vi "RT Loop - RSI Low Speed.vi"(11 "Message Queue":refnum<queue>) -> ()   [LabVIEW 2018]
doc: "This RSI Low Speed Loop VI acquires temperature data and digital inputs, and updates digital outputs."
uses:
  support/Message Queue/Message Cluster.ctl
  <vilib>/Platform/TimedLoop/XDataNode/timing_clust.ctl
  <vilib>/Platform/TimedLoop/XDataNode/nitl_modes.ctl
  <vilib>/Platform/TimedLoop/XDataNode/wakeup.ctl
  controls/Control State.ctl
  <vilib>/Platform/TimedLoop/XDataNode/loadnilvce.vi
  <vilib>/Platform/TimedLoop/XDataNode/XDataNode.xnode
  <vilib>/Platform/TimedLoop/XDataNode/XDNodeRunTimeDep.lvlib
  support/Message Queue/Message Queue.lvlib
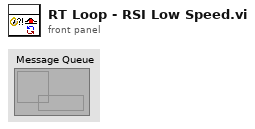
[diagram p1: front panel]
types:
  T1 = typedef "XDNodeRunTimeDep.lvlib/timing_clust.ctl" = cluster{"Expected End [f-1]":u64, "Actual End [f-1]":u64, "Finished Late? [f-1]":bool, "Expected End [i-1]":u64, "Actual End [i-1]":u64, "Finished Late? [i-1]":bool, "Expected Start [i]":u64, "Actual Start [i]":u64, "Expected Start [f]":u64, "Actual Start [f]":u64, "Source Name":string, "Structure Name":string, "Period":i64, "Deadline":i64, "Offset":i64, "Start":i64, "Priority":i32, "Timeout":i32, "Mode":T2, "Wakeup Reason":T3, "Error":errorcluster, "Source Type":string, "Secondary Source Type":string, "Global End Time":u64, "Global Start Time":u64, "Frame Duration":u64, "Iteration Duration":u64, "Assigned CPU":i32, "I/O Scan Engine Mode":u32}
  T2 = typedef "XDNodeRunTimeDep.lvlib/nitl_modes.ctl" = enum32{"No Change", "Process missed periods, maintain original phase", "Discard missed periods, maintain original phase", "Process missed periods, ignore original phase", "Discard missed periods, ignore original phase"}
  T3 = typedef "XDNodeRunTimeDep.lvlib/wakeup.ctl" = enum32{"Normal", "Aborted", "Asynchronous wakeup", "Timing source error", "Timed loop error", "Timeout"}
  T4 = typedef "Control State.ctl" = enum16{"Safe State", "Control (PID)"}
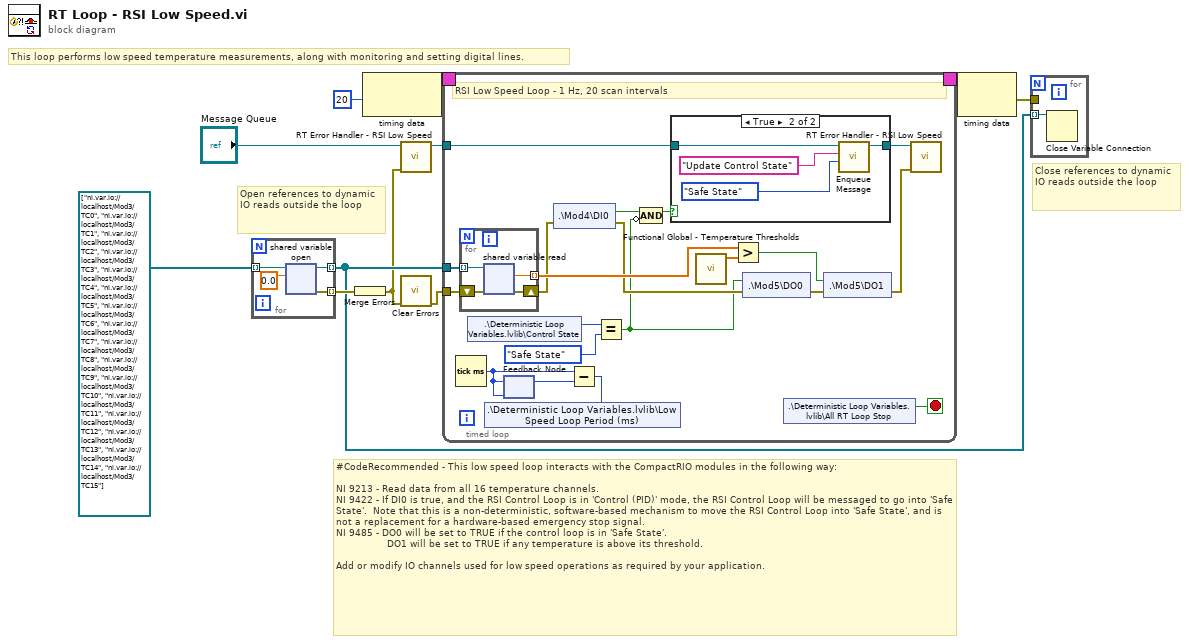
[diagram p0: block diagram]
diagram:
  # "Close references to dynamic IO reads outside the loop"
  # "Open references to dynamic IO reads outside the loop"
  # "#CodeRecommended - This low speed loop interacts with the CompactRIO modules in the following way:\n\nNI 9213 - Read data from all 16 temperature channels.\nNI 9422 - If DI0 is true, and the RSI Control Loop is in 'Control (PID)' mode, the RSI Control Loop will be messaged to go into 'Safe State'.  Note that this is a non-deterministic, software-based mechanism to move the RSI Control Loop into 'Safe State', and is not a replacement for a hardware-based emergency stop signal.\nNI 9485 - DO0 will be set to TRUE if the control loop is in 'Safe State'.\n                 DO1 will be set to TRUE if any temperature is above its threshold.\n\nAdd or modify IO channels used for low speed operations as required by your application."
  # "This loop performs low speed temperature measurements, along with monitoring and setting digital lines."
  n1 = for {
    tunnel: refnum<k21>[] ["ni.var.io://localhost/Mod3/TC0", "ni.var.io://localhost/Mod3/TC1", "ni.var.io://localhost/Mod3/TC2", "ni.var.io://localhost/Mod3/TC3", "ni.var.io://localhost/Mod3/TC4", "ni.var.io://localhost/Mod3/TC5", "ni.var.io://localhost/Mod3/TC6", "ni.var.io://localhost/Mod3/TC7", "ni.var.io://localhost/Mod3/TC8", "ni.var.io://localhost/Mod3/TC9", "ni.var.io://localhost/Mod3/TC10", "ni.var.io://localhost/Mod3/TC11", "ni.var.io://localhost/Mod3/TC12", "ni.var.io://localhost/Mod3/TC13", "ni.var.io://localhost/Mod3/TC14", "ni.var.io://localhost/Mod3/TC15"] -> [w15] mode=indexing
    tunnel: [w14] -> w4 mode=indexing
    tunnel: [w12] -> w6 mode=indexing
    n2 = shared-variable-open(w15, 0.0) -> (w14:refnum<k21>, w12:errorcluster)  [unwired: 2 in]
  }
  n3 = Merge Errors(w6) -> (w2:errorcluster)
  n4 = node-c288(i64 20 ("Period")) -> (w11:T1)
  n5 = call "RT Error Handler - RSI Low Speed.vi"("error in (no error)"=w2, "Message Queue"="Message Queue") -> ("dup Message Queue"=w7:refnum<queue>)  [unwired: 8 in, 1 out]
  n6 = call <vilib>:"Clear Errors.vi"("error in (no error)"=w2) -> ("error out"=w1:errorcluster)  [unwired: 5 in, 1 out]
  n7 = timed-loop {
    timing: w11 -> [_]
    timing-out: [_] -> w10
    tunnel: w7 -> [w33]
    tunnel: w4 -> [w24]
    tunnel: w1 -> [w19]
    stop <- w18 stop-if-true
    # "RSI Low Speed Loop - 1 Hz, 20 scan intervals"
    n8 = Tick Count (ms)() -> (millisecond timer value=w35:u32)
    n9 = for {
      tunnel: [w44] -> w26 mode=indexing
      tunnel: w24 -> [w43] mode=indexing
      shift-right: [w42] -> w23
      shift-left: w19 -> [w41]
      n10 = shared-variable-read(w43, w41) -> (w42:errorcluster, w44:dbl)  [unwired: 2 out]
    }
    n11 = shared-variable ".\\Deterministic Loop Variables.lvlib\\Control State"() -> (w16:T4)  [unwired: 1 in, 1 out]
    n12 = feedback #1(w35) -> (w34:u32)
    n13 = feedback-in #1(w35) -> ()
    n14 = shared-variable ".\\Mod4\\DI0"(error in=w23) -> (w32:bool, error out=w22:errorcluster)
    n15 = Subtract(x=w35, y=w34) -> (x-y=w17:u32)
    n16 = shared-variable ".\\Deterministic Loop Variables.lvlib\\Low Speed Loop Period (ms)"(w17) -> ()  [unwired: 1 in, 1 out]
    n17 = Equal?(x=w16, y=Control_State."Safe State" ("FPGA State")) -> (x = y?=w20:bool)
    n18 = Compound Arithmetic op=AND(w32, invert w20) -> (w21:bool)
    n19 = case shown="True" w21 {
      tunnel: w33 -> [w36 w40]
      tunnel: [w36 w39] -> w31
      frame False {
      }
      frame True {
        n20 = call "Enqueue Message.vi"("Message Data"=Control_State."Safe State" ("FPGA State"), "Message"="Update Control State", "Message Queue"=w40) -> ("dup Message Queue"=w39:refnum<queue>)  [unwired: 7 in, 1 out]
      }
    }
    n21 = call "Functional Global - Temperature Thresholds.vi"() -> ("Temperature Thresholds out"=w27:dbl[])  [unwired: 11 in]
    n22 = Greater?(x=w26, y=w27) -> (0:w25:bool)
    n23 = shared-variable ".\\Mod5\\DO0"(w20, error in=w22) -> (error out=w29:errorcluster)
    n24 = shared-variable ".\\Deterministic Loop Variables.lvlib\\All RT Loop Stop"() -> (w18:bool)  [unwired: 1 in, 1 out]
    n25 = shared-variable ".\\Mod5\\DO1"(w25, error in=w29) -> (error out=w28:errorcluster)
    n26 = call "RT Error Handler - RSI Low Speed.vi"("error in (no error)"=w28, "Message Queue"=w31) -> ()  [unwired: 8 in, 2 out]
  }
  n27 = node-c288(w10) -> (w5:errorcluster)
  n28 = for {
    tunnel: w5 -> [_]
    tunnel: w4 -> [w47] mode=indexing
    n29 = Close Variable Connection(11:w47) -> ()  [unwired: 1 in, 1 out]
  }
